vi "access table insert sqlite.vi"(8 "error in (no error)":errorcluster, 9 "Password":string, 10 "table":string, 11 "路径":path) -> (0 "错误输出":errorcluster, 3 "条数":i32)   [LabVIEW 2016]
uses:
  <vilib>/addons/database/Connection.llb/DB Tools Open Connec (String).vi
  <vilib>/addons/database/NI_Database_API.lvlib
  SQLite/SQLite Lib.lvlib
  Access/Access Lib.lvlib
panel:
  out "名称":string
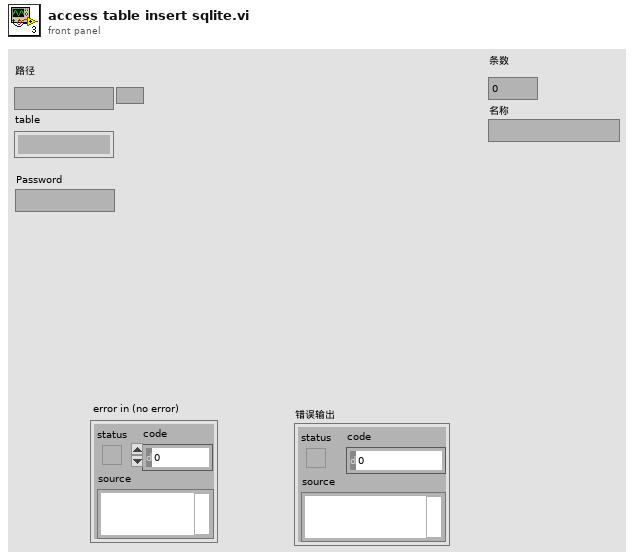
[diagram p1: front panel]
types:
  T1 = cluster{"columns外部输入":bool, "columns input":string[]}
  T2 = typedef "NI_Database_API.lvlib/Conn ObjectReference.ctl" = refnum<k1>
  T3 = typedef "NI_Database_API.lvlib/DB Tools DataTypes.ctl" = enum16{"String", "Long (I32)", "Single (SGL)", "Double (DBL)", "Date/Time", "Binary"}
  T4 = cluster{"name":string, "database data type":T3, "defined size":i32}[]
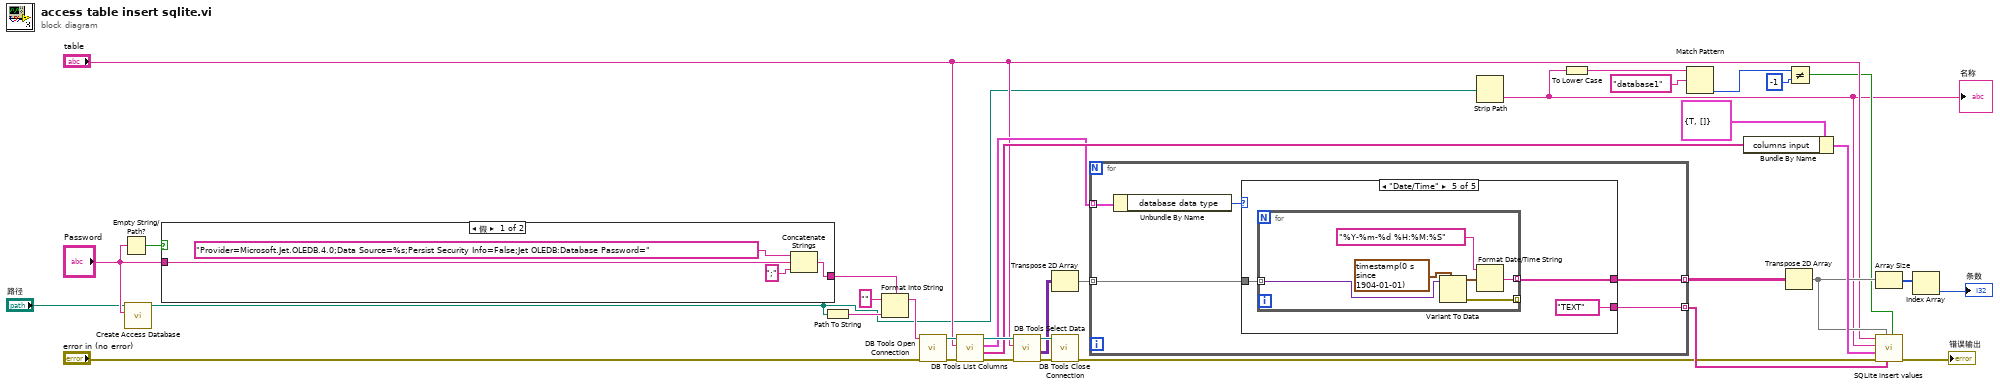
[diagram p0: block diagram]
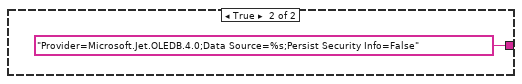
[diagram p2: hidden frame]
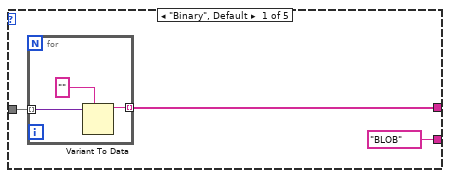
[diagram p3: hidden frame]
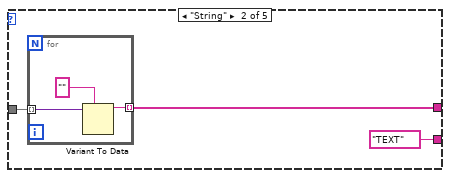
[diagram p4: hidden frame]
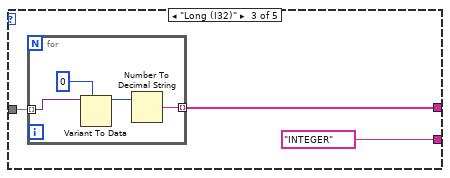
[diagram p5: hidden frame]
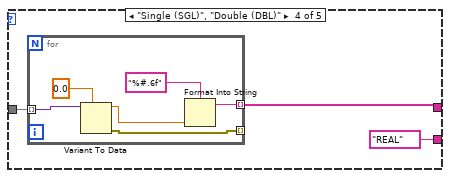
[diagram p6: hidden frame]
diagram:
  n1 = Empty String/Path?(string/path="Password") -> (empty?=w8:bool)
  n2 = call "Create Access Database.vi"("Password"="Password", "路径"="路径") -> ("路径 out"=w1:path)  [unwired: 8 in, 1 out]
  n3 = case shown="假" w8 {
    tunnel: [w36 "Provider=Microsoft.Jet.OLEDB.4.0;Data Source=%s;Persist Security Info=False" ("格式字符串")] -> w6
    tunnel: "Password" -> [w39 _]
    frame False {
      n4 = Concatenate Strings("Provider=Microsoft.Jet.OLEDB.4.0;Data Source=%s;Persist Security Info=False;Jet OLEDB:Database Password=" ("格式字符串"), w39, ";" ("字符串")) -> (w36:string)
    }
    frame True {
    }
  }
  n5 = Path To String(path=w1) -> (string=w4:string)
  n6 = Format Into String(format string=w6, initial string="" ("初始字符串"), w4) -> (resulting string=w2:string)  [unwired: 1 in, 1 out]
  n7 = call-poly <vilib>:"DB Tools Open Connection.vi"("error in (no error)"="error in (no error)", "connection information"=w2) -> ("error out"=w31:errorcluster, "connection reference"=w35:T2)  [unwired: 6 in]
  n8 = call <vilib>:"DB Tools List Columns.vi"("error in (no error)"=w31, "table"="table", "connection reference"=w35) -> ("error out"=w30:errorcluster, "columns"=w27:string[], "column information"=w26:T4, "connection reference out"=w32:T2)  [unwired: 1 in]
  n9 = call <vilib>:"DB Tools Select Data.vi"("error in (no error)"=w30, "table"="table", "connection reference"=w32) -> ("error out"=w33:errorcluster, "data"=w24:variant[][], "connection reference out"=w34:T2)  [unwired: 3 in]
  n10 = Transpose 2D Array(2D array=w24) -> (transposed array=w23:variant[][])
  n11 = call <vilib>:"DB Tools Close Connection.vi"("error in (no error)"=w33, "connection reference"=w34) -> ("error out"=w21:errorcluster)  [unwired: 5 in]
  n12 = for {
    tunnel: w26 -> [w45] mode=indexing
    tunnel: [w43] -> w25 mode=indexing
    tunnel: w23 -> [w42] mode=indexing
    tunnel: [w41] -> w22 mode=indexing
    n13 = Unbundle By Name(w45) -> ("database data type"=w44:T3)
    n14 = case shown="\"Date/Time\"" w44 {
      tunnel: ["BLOB" ("组合框") "TEXT" ("组合框") "INTEGER" ("组合框") "REAL" ("组合框") "TEXT" ("组合框")] -> w43
      tunnel: w42 -> [w47 w53 w59 w66 w75]
      tunnel: [w46 w52 w58 w65 w74] -> w41
      frame "Binary", Default {
        n15 = for {
          tunnel: w47 -> [w50] mode=indexing
          tunnel: [w49] -> w46 mode=indexing
          n16 = Variant To Data(type="", Variant=w50) -> (data=w49:string)  [unwired: 1 in, 1 out]
        }
      }
      frame "String" {
        n17 = for {
          tunnel: w53 -> [w56] mode=indexing
          tunnel: [w55] -> w52 mode=indexing
          n18 = Variant To Data(type="", Variant=w56) -> (data=w55:string)  [unwired: 1 in, 1 out]
        }
      }
      frame "Long (I32)" {
        n19 = for {
          tunnel: w59 -> [w62] mode=indexing
          tunnel: [w61] -> w58 mode=indexing
          n20 = Variant To Data(type=0, Variant=w62) -> (data=w64:i32)  [unwired: 1 in, 1 out]
          n21 = Number To Decimal String(number=w64) -> (decimal integer string=w61:string)  [unwired: 1 in]
        }
      }
      frame "Single (SGL)", "Double (DBL)" {
        n22 = for {
          tunnel: w66 -> [w70] mode=indexing
          tunnel: [w69] -> w65 mode=indexing
          tunnel: [w68] -> _ mode=indexing
          n23 = Variant To Data(type=sgl 0.0, Variant=w70) -> (data=w72:sgl, error out=w68:errorcluster)  [unwired: 1 in]
          n24 = Format Into String(format string="%#.6f" ("格式字符串"), w72) -> (resulting string=w69:string)  [unwired: 2 in, 1 out]
        }
      }
      frame "Date/Time" {
        n25 = for {
          tunnel: w75 -> [w80] mode=indexing
          tunnel: [w78] -> w74 mode=indexing
          tunnel: [w77] -> _ mode=indexing
          n26 = Variant To Data(type=timestamp(0 s since 1904-01-01) ("时间标识"), Variant=w80) -> (data=w79:timestamp, error out=w77:errorcluster)  [unwired: 1 in]
          n27 = Format Date/Time String(time format string (%c)="%Y-%m-%d %H:%M:%S" ("时间格式字符串(%c)"), seconds (now)=w79) -> (date/time string=w78:string)  [unwired: 1 in]
        }
      }
    }
  }
  n28 = Strip Path(path=w1) -> (name=w10:string)  [unwired: 1 out]
  "名称" <- w10
  n29 = To Lower Case(string=w10) -> (all lower case string=w9:string)
  n30 = Match Pattern(string=w9, regular expression="database1" ("正则表达式")) -> (offset past match=w13:i32)  [unwired: 1 in, 3 out]
  n31 = Bundle By Name(cluster=T1 {"columns外部输入"=TRUE, "columns input"=[]} ("columns外部输入"), "columns input"=w27) -> (w28:T1)
  n32 = Transpose 2D Array(2D array=w22) -> (transposed array=w18:string[][])
  n33 = Not Equal?(x=w13, y=-1) -> (x != y?=w11:bool)
  n34 = Array Size(array=w18) -> (size(s)=w17:i32[])
  n35 = call "SQLite insert values.vi"("是否创建唯一键"=w11, "columns  INFO"=w25, "数组"=w18, "错误输入（无错误）"=w21, "columns外部输入"=w28, "database"=w10, "Tabe Name"="table") -> ("错误输出"=→"错误输出":errorcluster)  [unwired: 4 in]
  n36 = Index Array(array=w17) -> (element=→"条数":i32)  [unwired: 1 in]
